vi "get_total_number_of_pixels_per_cycle.vi"(8 "error in (no error)":errorcluster, 11 "TrajectoryMG100122AODFrameScan in":refnum<class "TrajectoryMH100122AODRAPS.lvclass">) -> (0 "error out":errorcluster, 2 "total number of pixels per cycle":i32, 3 "TrajectoryMG100122AODFrameScan out":refnum<class "TrajectoryMH100122AODRAPS.lvclass">)   [LabVIEW 2010, in "TrajectoryMH100122AODRAPS.lvclass"]
uses:
  TrajectoryMH100122AODRAPS.lvclass
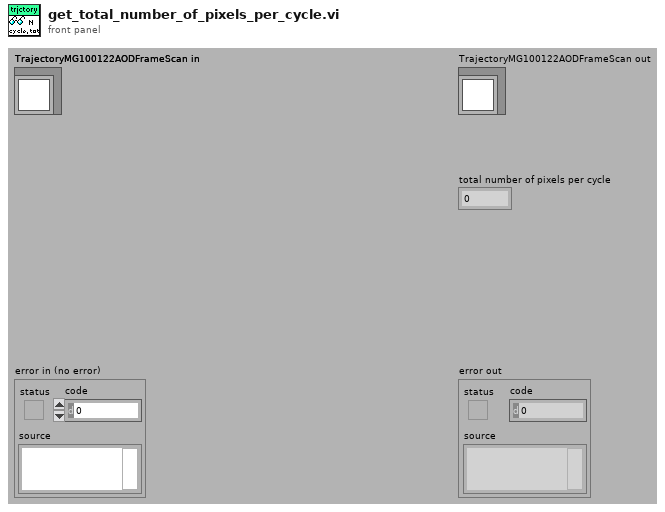
[diagram p1: front panel]
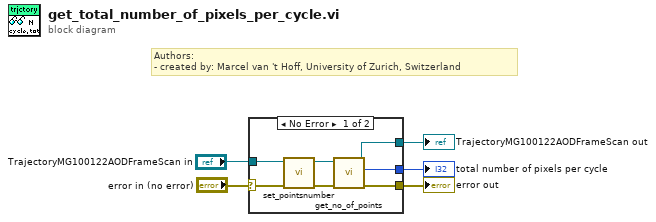
[diagram p0: block diagram]
diagram:
  # "Authors: \n- created by: Marcel van 't Hoff, University of Zurich, Switzerland"
  n1 = case shown="No Error" "error in (no error)" {
    selector: "error in (no error)" -> [w9 w13]
    tunnel: [w10 _] -> w5
    tunnel: "TrajectoryMG100122AODFrameScan in" -> [w7 w14]
    tunnel: [w11 w13] -> w3
    tunnel: [w12 w14] -> w1
    frame No Error {
      n2 = call-dynamic "set_pointsnumber.vi"("error in (no error)"=w9, "TrajectoryMH100122AODRAPS in"=w7) -> ("error out"=w8:errorcluster, "TrajectoryMH100122AODRAPS out"=w6:refnum<class "TrajectoryMH100122AODRAPS.lvclass">)  [unwired: 8 in]
      n3 = call-dynamic "get_no_of_points.vi"("error in (no error)"=w8, "TrajectoryMH100122AODRAPS in"=w6) -> ("error out"=w11:errorcluster, "no. of points"=w10:i64, "TrajectoryMH100122AODRAPS out"=w12:refnum<class "TrajectoryMH100122AODRAPS.lvclass">)  [unwired: 7 in]
    }
    frame Error {
    }
  }
  "error out" <- w3
  "TrajectoryMG100122AODFrameScan out" <- w1
  "total number of pixels per cycle" <- w5
